vi "Programmatically Create SV.vi"(10 "database":path=path "C:/Ehsan Temp Folder/TFS/LV/Data Logging with LabVIEW/Database/FromDDS.csv" caption="Database (.csv) - \";\" separated", 11 "Project Address":path=path "C:/Ehsan Temp Folder/TFS/LV/Data Logging with LabVIEW/qq.lvproj") -> ()   [LabVIEW 2014]
uses:
  TypeDef/Q1 Create SV.ctl
  <vilib>/Utility/file.llb/Read From Spreadsheet File (string).vi
  <vilib>/Platform/browser.llb/Open URL in Default Browser (path).vi
  <vilib>/Utility/file.llb/Write To Spreadsheet File (string).vi
panel:
  in  "lib name":bool
  in  "Library Name":string="SV Library" caption="Library Name (Save As)"
  in  "save":bool
  in  "Bind":bool
  in  "Create":bool
  in  "exit":bool
  in  "initialize":bool
  out "Database":string[][](array[string])
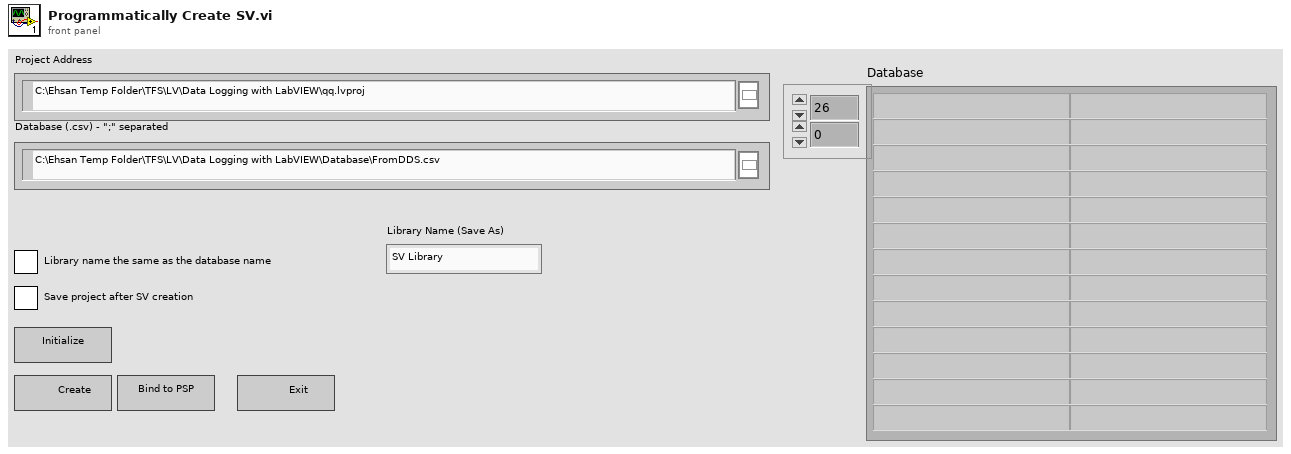
[diagram p1: front panel]
types:
  T1 = enum8{"Enabled", "Disabled", "Disabled and Grayed Out"}
  T2 = typedef "Q1 Create SV.ctl" = cluster{"State":enum16{"Initialize", "Idle", "Prepare", "Create", "Save Library", "Bind SV", "Exit", "Error", "Save Project", "Check Library Name"}, "Data":variant}
  T3 = enum16{"Initialize", "Idle", "Prepare", "Create", "Save Library", "Bind SV", "Exit", "Error", "Save Project", "Check Library Name"}
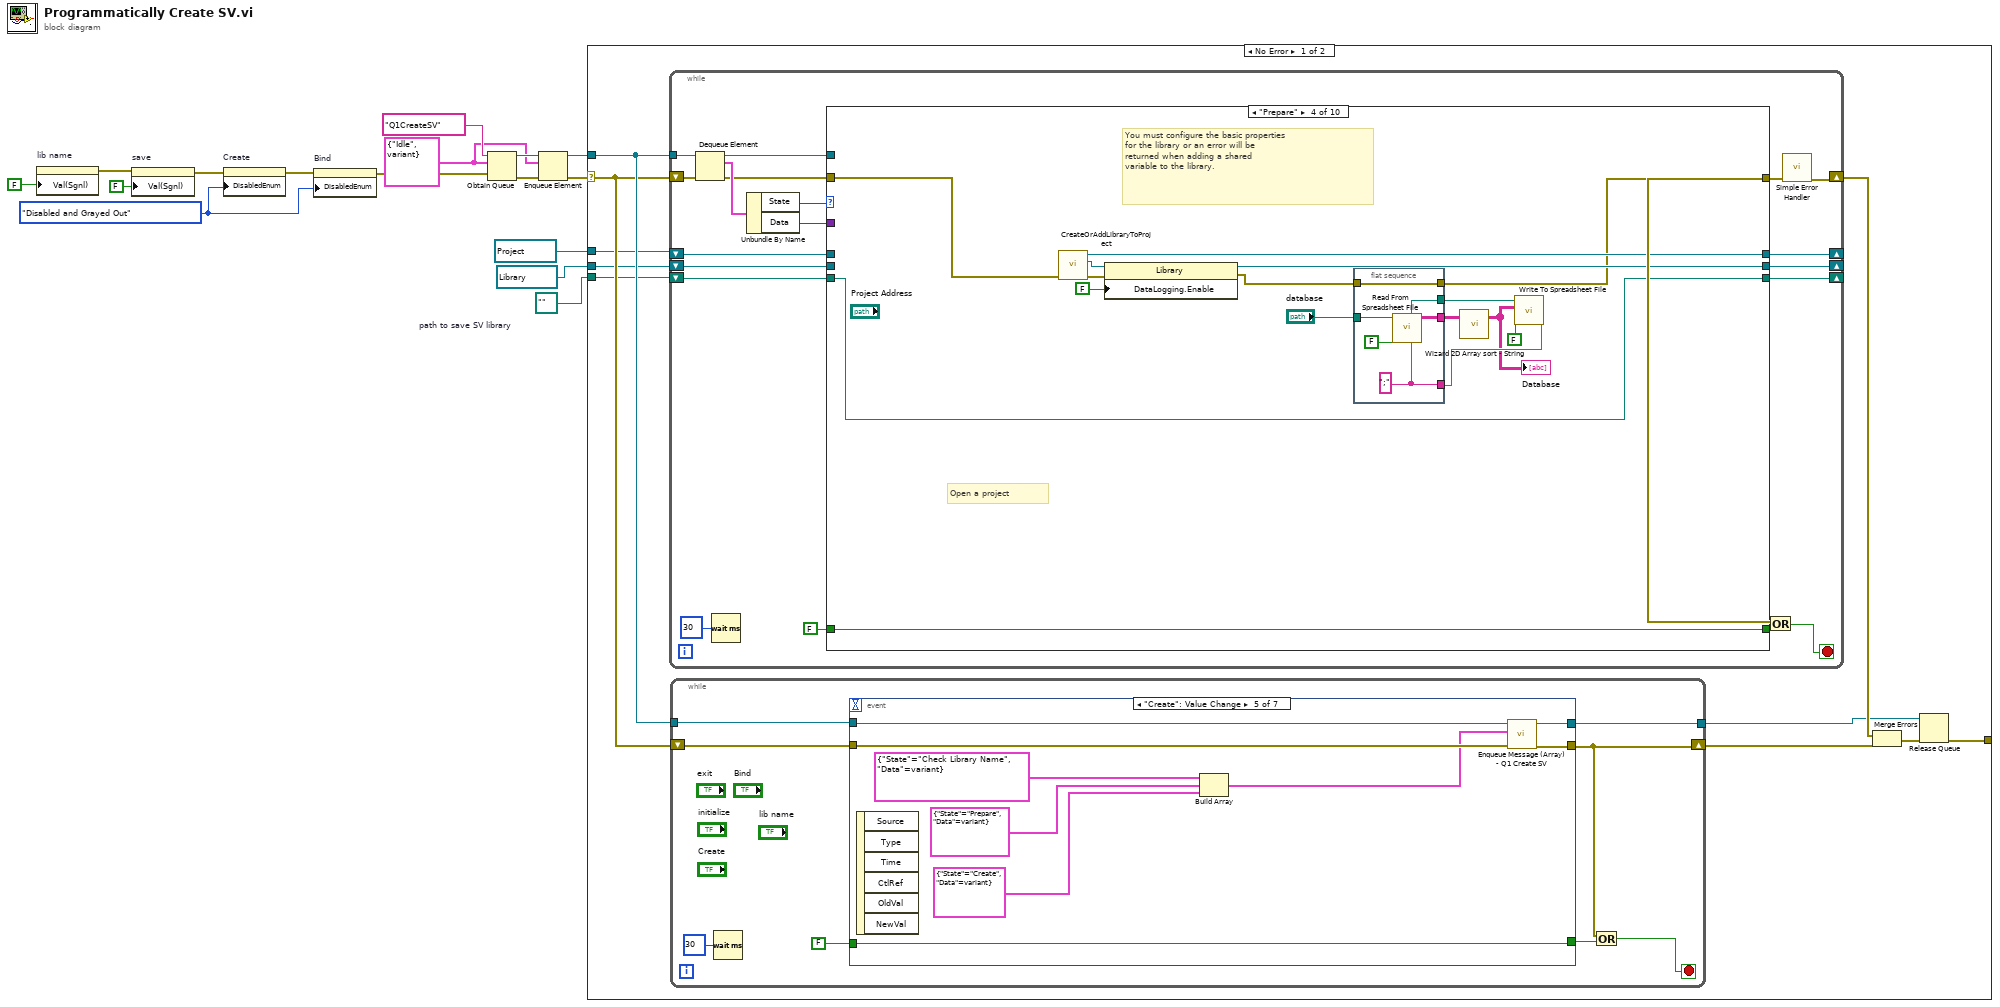
[diagram p0: block diagram]
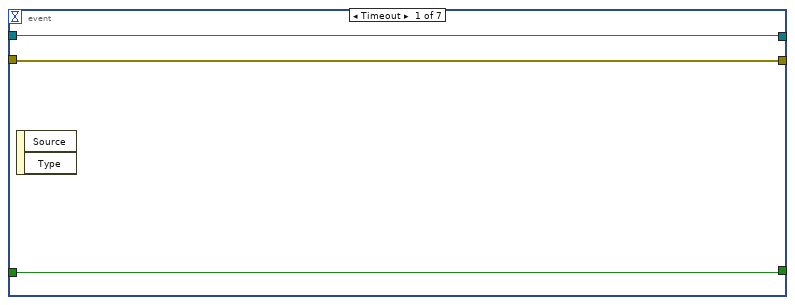
[diagram p2: hidden frame]
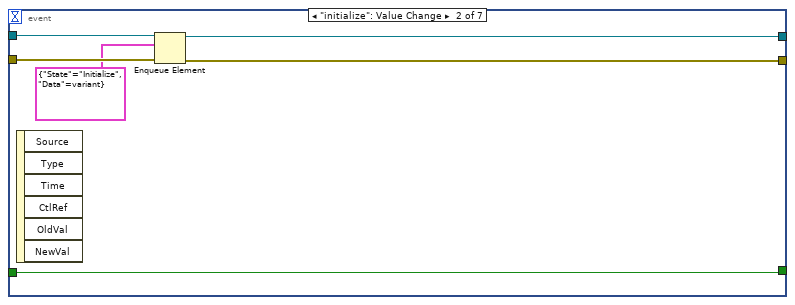
[diagram p3: hidden frame]
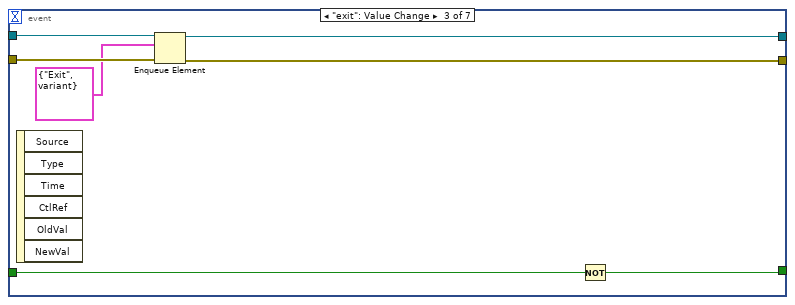
[diagram p4: hidden frame]
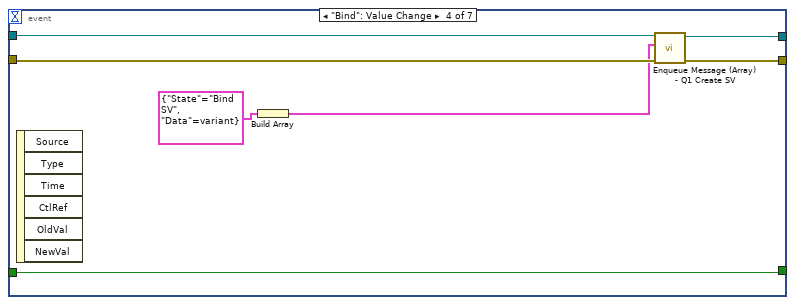
[diagram p5: hidden frame]
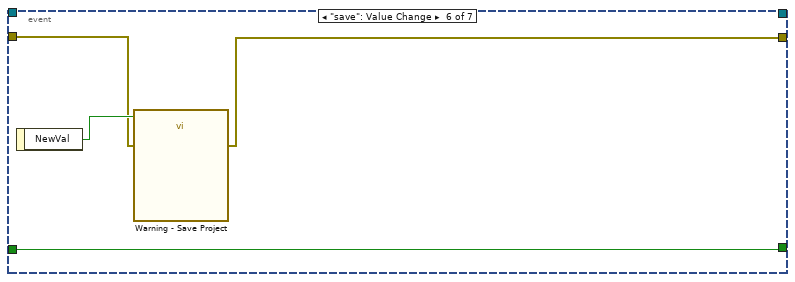
[diagram p6: hidden frame]
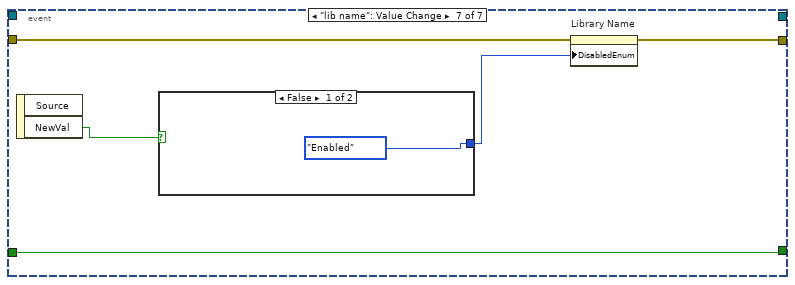
[diagram p7: hidden frame]
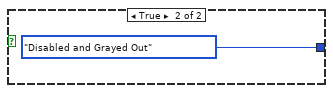
[diagram p8: hidden frame]
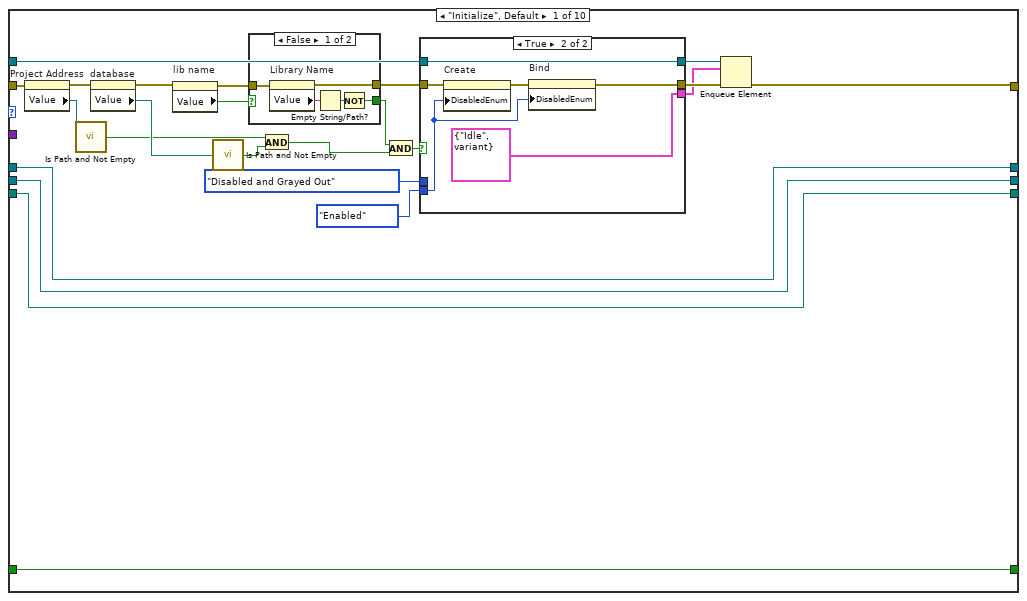
[diagram p9: hidden frame]
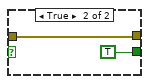
[diagram p10: hidden frame]
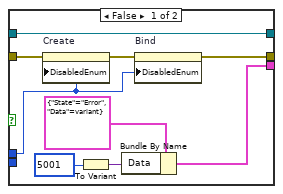
[diagram p11: hidden frame]
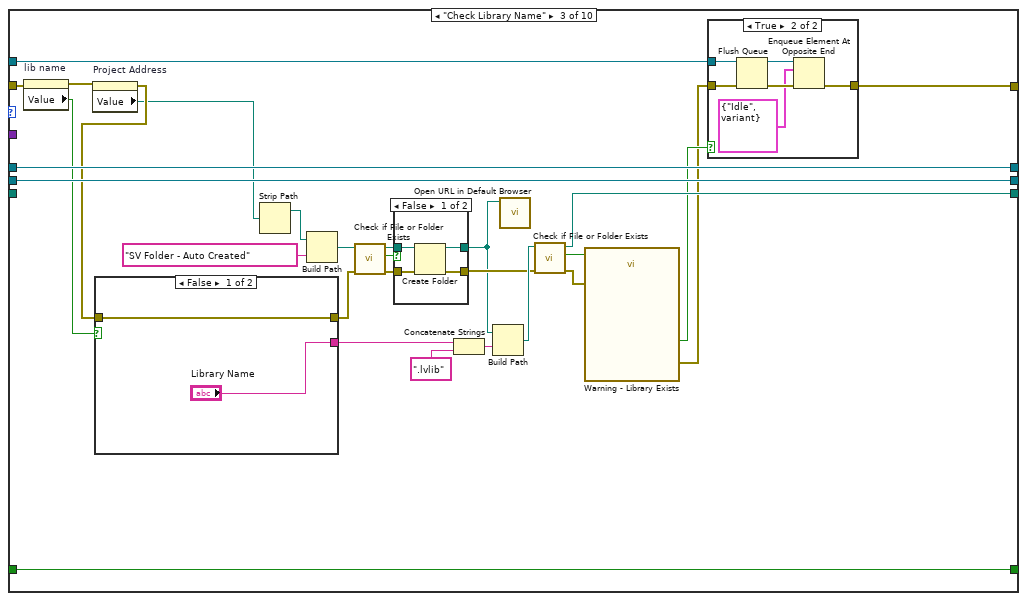
[diagram p13: hidden frame]
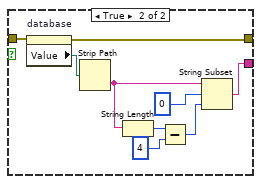
[diagram p14: hidden frame]
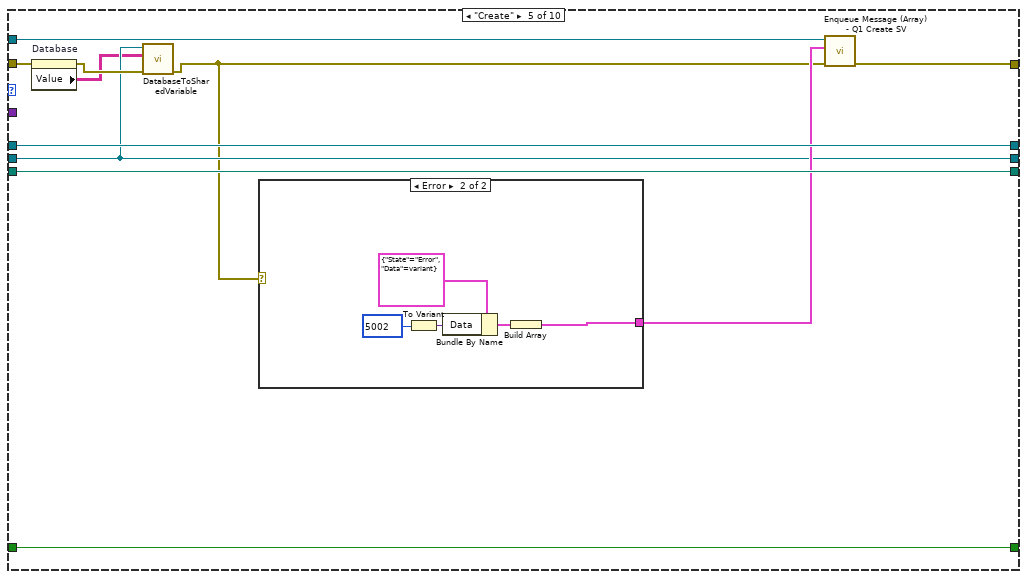
[diagram p17: hidden frame]
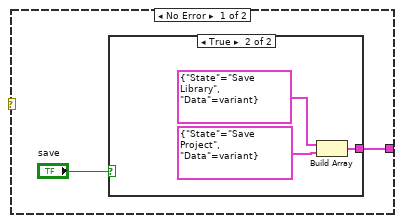
[diagram p18: hidden frame]
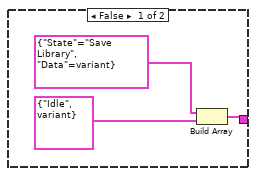
[diagram p19: hidden frame]
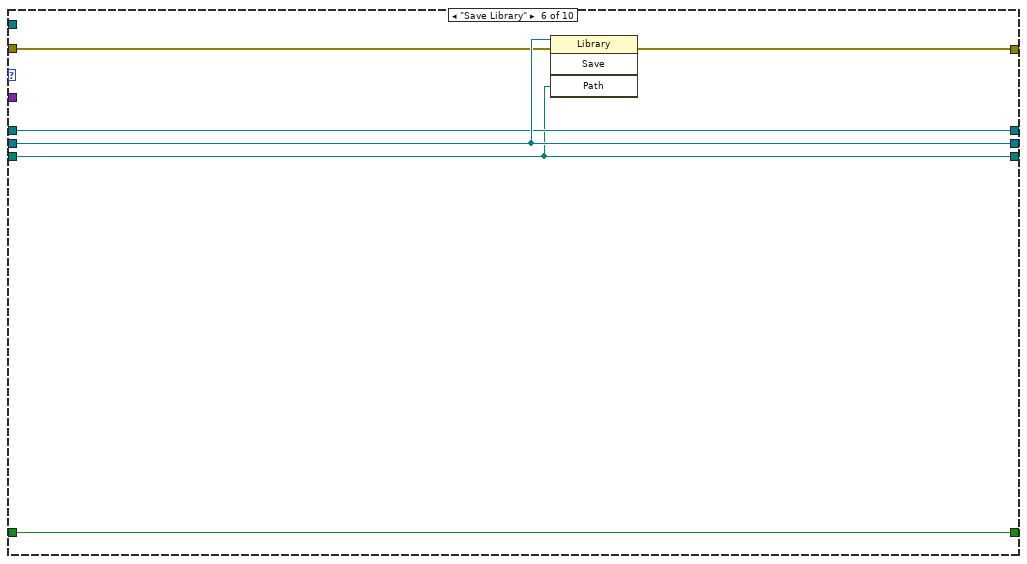
[diagram p20: hidden frame]
diagram:
  w6 = T1."Disabled and Grayed Out" ("Disabled")
  w8 = path ""  # path to save SV library
  w13 = T2 {"State"=enum."Idle", "Data"=variant}
  n1 = property on="lib name" class="Bool (strict)"("Val(Sgnl)"=FALSE ("Value (Signaling)")) -> (error out=w1:errorcluster)  [unwired: 2 in, 1 out]
  n2 = property on="save" class="Bool (strict)"(error in=w1, "Val(Sgnl)"=FALSE ("Value (Signaling)")) -> (error out=w4:errorcluster)  [unwired: 1 in, 1 out]
  n3 = property on="Create" class="Bool"(error in=w4, "DisabledEnum"=w6) -> (error out=w7:errorcluster)  [unwired: 1 in, 1 out]
  n4 = property on="Bind" class="Bool"(error in=w7, "DisabledEnum"=w6) -> (error out=w5:errorcluster)  [unwired: 1 in, 1 out]
  n5 = Obtain Queue(name (unnamed)="Q1CreateSV", element data type=w13, error in (no error)=w5) -> (queue out=w15:refnum<queue>, error out=w14:errorcluster)  [unwired: 2 in, 1 out]
  n6 = Enqueue Element(queue=w15, element=w13, error in (no error)=w14) -> (queue out=w11:refnum<queue>, error out=w12:errorcluster)  [unwired: 1 in, 1 out]
  n7 = case shown="No Error" w12 {
    selector: w12 -> [w25 w312]
    tunnel: w11 -> [w26 _]
    tunnel: refnum<vi> refnum ("Project Reference Out") -> [w24 _]
    tunnel: [w19 w312] -> _
    tunnel: refnum<vi> refnum ("Library Reference Out") -> [w18 _]
    tunnel: w8 -> [w17 _]
    frame No Error {
      n8 = while {
        tunnel: w26 -> [w95]
        shift-right: [w79] -> w22
        shift-left: w25 -> [w96]
        shift-right: [w86] -> _
        shift-left: w24 -> [w85]
        shift-right: [w84] -> _
        shift-left: w18 -> [w83]
        shift-right: [w82] -> _
        shift-left: w17 -> [w81]
        stop <- w88 stop-if-true
        n9 = Dequeue Element(queue=w95, error in (no error)=w96) -> (queue out=w91:refnum<queue>, element=w94:T2, error out=w80:errorcluster)  [unwired: 1 in, 1 out]
        n10 = Wait (ms)(milliseconds to wait=u32 30) -> ()  [unwired: 1 out]
        n11 = Unbundle By Name(w94) -> ("State"=w93:T3, "Data"=w92:variant)
        n12 = case shown="\"Prepare\"" w93 {
          tunnel: w92 -> [_ _ _ _ _ _ _ _ _ w310]
          tunnel: w91 -> [w108 _ w156 _ w229 _ _ w265 w290 w300]
          tunnel: FALSE -> [w120 w147 w175 w215 w232 w251 w259 w271 w289 w311]
          tunnel: [w120 w147 w175 w215 w232 w251 w259 w271 w288 w311] -> w89
          tunnel: [w105 w146 w174 w211 w231 w249 w255 w270 w279 w303] -> w86
          tunnel: w85 -> [w105 w146 w174 _ w231 w249 w255 w270 w279 w303]
          tunnel: [w104 w145 w173 w210 w224 w250 w256 w269 w284 w302] -> w84
          tunnel: w83 -> [w104 w145 w173 _ w224 w250 w256 w269 w284 w302]
          tunnel: [w103 w144 w160 w208 w230 w247 w258 w268 w287 w301] -> w82
          tunnel: w81 -> [w103 w144 _ w208 w230 w247 w258 w268 w287 w301]
          tunnel: [w102 w143 w157 w206 w227 w248 w253 w263 w286 w297] -> w78
          tunnel: w80 -> [w101 w143 w153 w202 w226 w246 w252 w261 w285 _]
          frame "Initialize", Default {
            n13 = property on="Project Address" class="Path"(error in=w101) -> (error out=w119:errorcluster, "Value"=w118:path)  [unwired: 1 in, 1 out]
            n14 = call <vilib>:"Is Path and Not Empty.vi"("path"=w118) -> ("Is Path and Not Empty?"=w115:bool)  [unwired: 4 in]
            n15 = property on="database" class="Path"(error in=w119) -> (error out=w100:errorcluster, "Value"=w117:path)  [unwired: 1 in, 1 out]
            n16 = property on="lib name" class="Bool (strict)"(error in=w100) -> (error out=w98:errorcluster, "Value"=w99:bool)  [unwired: 1 in, 1 out]
            n17 = call <vilib>:"Is Path and Not Empty.vi"("path"=w117) -> ("Is Path and Not Empty?"=w116:bool)  [unwired: 4 in]
            n18 = case shown="False" w99 {
              tunnel: [w124 TRUE] -> w114
              tunnel: w98 -> [w122 w127]
              tunnel: [w121 w127] -> w97
              frame False {
                n19 = property on="Library Name" class="Str"(error in=w122) -> (error out=w121:errorcluster, "Value"=w123:string)  [unwired: 1 in, 1 out]
                n20 = Empty String/Path?(string/path=w123) -> (empty?=w125:bool)
                n21 = Not(x=w125) -> (.not. x?=w124:bool)
              }
              frame True {
              }
            }
            n22 = And(x=w115, y=w116) -> (x .and. y?=w113:bool)
            n23 = And(x=w114, y=w113) -> (x .and. y?=w112:bool)
            n24 = case shown="True" w112 {
              tunnel: T1."Disabled and Grayed Out" ("Disabled") -> [w129 _]
              tunnel: T1."Enabled" ("Disabled") -> [_ w139]
              tunnel: [w133 T2 {"State"=enum."Idle", "Data"=variant}] -> w106
              tunnel: [w130 w138] -> w109
              tunnel: w108 -> [w132 w141]
              tunnel: [w132 w141] -> w107
              tunnel: w97 -> [w128 w137]
              frame False {
                n25 = property on="Create" class="Bool"(error in=w128, "DisabledEnum"=w129) -> (error out=w131:errorcluster)  [unwired: 1 in, 1 out]
                n26 = To Variant(anything=5001) -> (Variant=w134:variant)
                n27 = Bundle By Name(cluster=T2 {"State"=enum."Error", "Data"=variant}, "Data"=w134) -> (w133:T2)
                n28 = property on="Bind" class="Bool"(error in=w131, "DisabledEnum"=w129) -> (error out=w130:errorcluster)  [unwired: 1 in, 1 out]
              }
              frame True {
                n29 = property on="Create" class="Bool"(error in=w137, "DisabledEnum"=w139) -> (error out=w140:errorcluster)  [unwired: 1 in, 1 out]
                n30 = property on="Bind" class="Bool"(error in=w140, "DisabledEnum"=w139) -> (error out=w138:errorcluster)  [unwired: 1 in, 1 out]
              }
            }
            n31 = Enqueue Element(queue=w107, element=w106, error in (no error)=w109) -> (error out=w102:errorcluster)  [unwired: 1 in, 2 out]
          }
          frame "Idle" {
          }
          frame "Check Library Name" {
            n32 = property on="lib name" class="Bool (strict)"(error in=w153) -> (error out=w152:errorcluster, "Value"=w155:bool)  [unwired: 1 in, 1 out]
            n33 = property on="Project Address" class="Path"(error in=w152) -> (error out=w151:errorcluster, "Value"=w149:path)  [unwired: 1 in, 1 out]
            n34 = case shown="False" w155 {
              tunnel: ["Library Name" w183] -> w154
              tunnel: [w176 w185] -> w150
              tunnel: w151 -> [w176 w186]
              frame False {
              }
              frame True {
                n35 = property on="database" class="Path"(error in=w186) -> (error out=w185:errorcluster, "Value"=w184:path)  [unwired: 1 in, 1 out]
                n36 = Strip Path(path=w184) -> (name=w181:string)  [unwired: 1 out]
                n37 = String Length(string=w181) -> (length=w180:i32)
                n38 = Subtract(x=w180, y=4) -> (x-y=w178:i32)
                n39 = String Subset(string=w181, offset (0)=0, length (rest)=w178) -> (substring=w183:string)
              }
            }
            n40 = Strip Path(path=w149) -> (stripped path=w172:path)  [unwired: 1 out]
            n41 = Build Path(base path=w172, name or relative path="SV Folder - Auto Created") -> (appended path=w170:path)
            n42 = call <vilib>:"Check if File or Folder Exists.vi"("error in (no error)"=w150, "path"=w170) -> ("error out"=w169:errorcluster, "file or folder exists?"=w168:bool, "dup path"=w167:path)  [unwired: 7 in]
            n43 = case shown="False" w168 {
              tunnel: [w197 w198] -> w148
              tunnel: [w195 w199] -> w163
              tunnel: w169 -> [w196 w199]
              tunnel: w167 -> [w194 w198]
              frame False {
                n44 = Create Folder(path (use dialog)=w194, error in=w196) -> (created path=w197:path, error out=w195:errorcluster)  [unwired: 1 in, 1 out]
              }
              frame True {
              }
            }
            n45 = Concatenate Strings(w154, ".lvlib" ("string")) -> (w165:string)
            n46 = Build Path(base path=w148, name or relative path=w165) -> (appended path=w164:path)
            n47 = call-poly <vilib>:"Open URL in Default Browser.vi"("path"=w148) -> ()  [unwired: 5 in, 2 out]
            n48 = call <vilib>:"Check if File or Folder Exists.vi"("error in (no error)"=w163, "path"=w164) -> ("error out"=w162:errorcluster, "file or folder exists?"=w161:bool, "dup path"=w160:path)  [unwired: 7 in]
            n49 = call "Warning - Library Exists"("Enable"=w161, "error in (no error)"=w162) -> ("Stop"=w159:bool, "error out"=w158:errorcluster)  [unwired: 16 in]
            n50 = case shown="True" w159 {
              tunnel: [w187 w190] -> w157
              tunnel: w158 -> [w187 w189]
              tunnel: w156 -> [_ w188]
              frame False {
              }
              frame True {
                n51 = Flush Queue(queue=w188, error in (no error)=w189) -> (queue out=w193:refnum<queue>, error out=w192:errorcluster)  [unwired: 1 out]
                n52 = Enqueue Element At Opposite End(queue=w193, element=T2 {"State"=enum."Idle", "Data"=variant}, error in (no error)=w192) -> (error out=w190:errorcluster)  [unwired: 1 in, 2 out]
              }
            }
          }
          frame "Prepare" {
            # "Open a project"
            # "You must configure the basic properties\nfor the library or an error will be\nreturned when adding a shared\nvariable to the library."
            n53 = call <vilib>:"CreateOrAddLibraryToProject.vi"("error in (no error)"=w202) -> ("error out"=w213:errorcluster, "Library Reference Out"=w212:refnum<vi>, "Project Reference Out"=w211:refnum<vi>)  [unwired: 8 in]
            n54 = property class="Library"(reference=w212, error in=w213, "DataLogging.Enable"=FALSE ("DataLogging:Enable")) -> (reference out=w210:refnum<vi>, error out=w207:errorcluster)
            n55 = flat-sequence {
              tunnel: "database" -> [w220]
              tunnel: [w219] -> w201
              tunnel: w207 -> [w218]
              tunnel: [w218] -> w206
              tunnel: [w217] -> w205
              tunnel: [w216] -> w204
              frame #0 {
                w216 = ";" ("delimiter (\\t)")
                n56 = call-poly <vilib>:"Read From Spreadsheet File.vi"("delimiter (\\t)"=w216, "transpose (no:F)"=FALSE, "file path (dialog if empty)"=w220) -> ("all rows"=w219:string[][], "new file path (Not A Path if cancelled)"=w217:path)  [unwired: 4 in, 3 out]
              }
            }
            n57 = call "Wizard 2D Array sort - String.vi"("Array In"=w201) -> ("Array Out"=w200:string[][])  [unwired: 1 in, 1 out]
            "Database" <- w200
            n58 = call-poly <vilib>:"Write To Spreadsheet File.vi"("delimiter (\\t)"=w204, "append to file? (new file:F)"=FALSE, "2D data"=w200, "file path (dialog if empty)"=w205) -> ()  [unwired: 4 in, 1 out]
          }
          frame "Create" {
            n59 = property on="Database" class="Arr (strict)"(error in=w226) -> (error out=w225:errorcluster, "Value"=w223:string[][])  [unwired: 1 in, 1 out]
            n60 = call "DatabaseToSharedVariable.vi"("error in"=w225, 10:w223, "Library in"=w224) -> ("error out"=w222:errorcluster)  [unwired: 6 in, 2 out]
            n61 = case shown="Error" w222 {
              tunnel: [w234 w242] -> w228
              frame No Error {
                n62 = case shown="True" "save" {
                  tunnel: [w236 w238] -> w234
                  frame False {
                    n63 = Build Array(T2 {"State"=enum."Save Library", "Data"=variant}, T2 {"State"=enum."Idle", "Data"=variant}) -> (w236:T2[])
                  }
                  frame True {
                    n64 = Build Array(T2 {"State"=enum."Save Library", "Data"=variant}, T2 {"State"=enum."Save Project", "Data"=variant}) -> (w238:T2[])
                  }
                }
              }
              frame Error {
                n65 = To Variant(anything=5002) -> (Variant=w243:variant)
                n66 = Bundle By Name(cluster=T2 {"State"=enum."Error", "Data"=variant}, "Data"=w243) -> (w241:T2)
                n67 = Build Array(w241) -> (w242:T2[])
              }
            }
            n68 = call "Enqueue Message (Array) - Q1 Create SV.vi"("error in (no error)"=w222, "Message Array"=w228, "Qin"=w229) -> ("error out"=w227:errorcluster)  [unwired: 7 in, 1 out]
          }
          frame "Save Library" {
            n69 = invoke class="Library" method="Save"(reference=w250, error in=w246, "Path"=w247) -> (error out=w248:errorcluster)  [unwired: 1 in, 3 out]
          }
          frame "Save Project" {
            n70 = property on="Project Address" class="Path"(error in=w252) -> (error out=w254:errorcluster, "Value"=w257:path)  [unwired: 1 in, 1 out]
            n71 = invoke class="Project" method="Save"(reference=w255, error in=w254, "Path"=w257) -> (error out=w253:errorcluster)  [unwired: 1 in, 3 out]
          }
          frame "Bind SV" {
            n72 = property on="Database" class="Arr (strict)"(error in=w261) -> (error out=w267:errorcluster, "Value"=w260:string[][])  [unwired: 1 in, 1 out]
            n73 = call "BindingVI.vi"("Library Path"=w268, "error in"=w267, "Binding info"=w260) -> ("error out"=w266:errorcluster, "Error status"=w264:bool)  [unwired: 7 in]
            n74 = case shown="True" w264 {
              tunnel: [w272 w275] -> w262
              frame False {
                n75 = Build Array(T2 {"State"=enum."Idle", "Data"=variant}) -> (w272:T2[])
              }
              frame True {
                n76 = To Variant(anything=5003) -> (Variant=w276:variant)
                n77 = Bundle By Name(cluster=T2 {"State"=enum."Error", "Data"=variant}, "Data"=w276) -> (w274:T2)
                n78 = Build Array(w274) -> (w275:T2[])
              }
            }
            n79 = call "Enqueue Message (Array) - Q1 Create SV.vi"("error in (no error)"=w266, "Message Array"=w262, "Qin"=w265) -> ("error out"=w263:errorcluster)  [unwired: 7 in, 1 out]
          }
          frame "Exit" {
            n80 = Flush Queue(queue=w290, error in (no error)=w285) -> (error out=w280:errorcluster)  [unwired: 2 out]
            n81 = Not A Number/Path/Refnum?(number/path/refnum=w279) -> (NaN/Path/Refnum?=w283:bool)
            n82 = Not A Number/Path/Refnum?(number/path/refnum=w284) -> (NaN/Path/Refnum?=w282:bool)
            n83 = Or(x=w283, y=w282) -> (x .or. y?=w281:bool)
            n84 = case shown="True" w281 {
              tunnel: w284 -> [w295 _]
              tunnel: [w294 w296] -> w286
              tunnel: w280 -> [w293 w296]
              tunnel: w279 -> [w291 _]
              frame False {
                n85 = Close Reference(reference=w291, error in (no error)=w293) -> (error out=w292:errorcluster)
                n86 = Close Reference(reference=w295, error in (no error)=w292) -> (error out=w294:errorcluster)
              }
              frame True {
              }
            }
            n87 = Not(x=w289) -> (.not. x?=w288:bool)
          }
          frame "Error" {
            n88 = Variant To Data(type=0, Variant=w310) -> (data=w308:i32, error out=w304:errorcluster)  [unwired: 1 in]
            n89 = call <vilib>:"General Error Handler.vi"("[error code] (0)"=w308, "[user-defined codes]"=i32[] [5001, 5002, 5003], "[user-defined descriptions]"=string[] ["Error occured at Initialize state. Project Address and/or Database Address may not be a path or may be empty. The Library Name may be empty.\n", "Error occured in Create state. The type of the shared variable is not known to this SubVI. ", "Error occured at Bind state. There is something wrong with database (binding server, binding library name, SV name) or with the library that is to be bound."], "[error source] (\" \")"="Automatically Creation of Shared Variables" ("[error source] (\" \")"), "error in (no error)"=w304) -> ("error out"=w299:errorcluster)  [unwired: 6 in, 4 out]
            n90 = Enqueue Element(queue=w300, element=T2 {"State"=enum."Idle", "Data"=variant}, error in (no error)=w299) -> (error out=w297:errorcluster)  [unwired: 1 in, 2 out]
          }
        }
        n91 = Or(x=w78, y=w89) -> (x .or. y?=w88:bool)
        n92 = call <vilib>:"Simple Error Handler.vi"("error in (no error)"=w78) -> ("error out"=w79:errorcluster)  [unwired: 4 in, 4 out]
      }
      n93 = while {
        tunnel: w26 -> [w34]
        shift-right: [w29] -> w23
        shift-left: w25 -> [w33]
        tunnel: [w27] -> w20
        stop <- w30 stop-if-true
        n94 = Wait (ms)(milliseconds to wait=u32 30) -> ()  [unwired: 1 out]
        n95 = event shown="[4] \"Create\": Value Change" {
          selector: _ -> [_ _ _ _ _ _ _]
          dyn-events: _ -> [_ _ _ _ _ _ _]
          timeout: _ -> [_ _ _ _ _ _ _]
          tunnel: w34 -> [w36 w43 w50 w53 w62 _ _]
          tunnel: w33 -> [w35 w42 w49 w54 w61 w68 w73]
          tunnel: FALSE -> [w37 w40 w46 w57 w66 w70 w75]
          tunnel: [w37 w40 w45 w57 w66 w70 w75] -> w31
          tunnel: [w35 w39 w47 w55 w60 w67 w72] -> w29
          tunnel: [w36 w38 w44 w56 w63 _ _] -> w27
          event Timeout {
            n96 = event-data() -> ()  [unwired: 1 in, 2 out]
          }
          event "initialize": Value Change {
            n97 = event-data() -> ()  [unwired: 1 in, 6 out]
            n98 = Enqueue Element(queue=w43, element=T2 {"State"=enum."Initialize", "Data"=variant}, error in (no error)=w42) -> (queue out=w38:refnum<queue>, error out=w39:errorcluster)  [unwired: 1 in, 1 out]
          }
          event "exit": Value Change {
            n99 = event-data() -> ()  [unwired: 1 in, 6 out]
            n100 = Enqueue Element(queue=w50, element=T2 {"State"=enum."Exit", "Data"=variant}, error in (no error)=w49) -> (queue out=w44:refnum<queue>, error out=w47:errorcluster)  [unwired: 1 in, 1 out]
            n101 = Not(x=w46) -> (.not. x?=w45:bool)
          }
          event "Bind": Value Change {
            n102 = event-data() -> ()  [unwired: 1 in, 6 out]
            n103 = Build Array(T2 {"State"=enum."Bind SV", "Data"=variant}) -> (w51:T2[])
            n104 = call "Enqueue Message (Array) - Q1 Create SV.vi"("error in (no error)"=w54, "Message Array"=w51, "Qin"=w53) -> ("error out"=w55:errorcluster, "Qout"=w56:refnum<queue>)  [unwired: 7 in]
          }
          event "Create": Value Change {
            n105 = event-data() -> ()  [unwired: 1 in, 6 out]
            n106 = Build Array(T2 {"State"=enum."Check Library Name", "Data"=variant}, T2 {"State"=enum."Prepare", "Data"=variant}, T2 {"State"=enum."Create", "Data"=variant}) -> (w59:T2[])
            n107 = call "Enqueue Message (Array) - Q1 Create SV.vi"("error in (no error)"=w61, "Message Array"=w59, "Qin"=w62) -> ("error out"=w60:errorcluster, "Qout"=w63:refnum<queue>)  [unwired: 7 in]
          }
          event "save": Value Change {
            n108 = event-data() -> ("NewVal"=w69:bool)  [unwired: 1 in]
            n109 = call "Warning - Save Project"("Enable"=w69, "error in (no error)"=w68) -> ("error out"=w67:errorcluster)  [unwired: 16 in, 1 out]
          }
          event "lib name": Value Change {
            n110 = event-data() -> ("NewVal"=w74:bool)  [unwired: 1 in, 1 out]
            n111 = case shown="False" w74 {
              tunnel: [T1."Enabled" ("Disabled") T1."Disabled and Grayed Out" ("Disabled")] -> w71
              frame False {
              }
              frame True {
              }
            }
            n112 = property on="Library Name" class="Str"(error in=w73, "DisabledEnum"=w71) -> (error out=w72:errorcluster)  [unwired: 1 in, 1 out]
          }
        }
        n113 = Or(x=w29, y=w31) -> (x .or. y?=w30:bool)
      }
      n114 = Merge Errors(w22, w23) -> (w21:errorcluster)
      n115 = Release Queue(queue=w20, error in (no error)=w21) -> (error out=w19:errorcluster)  [unwired: 1 in, 2 out]
    }
    frame Error {
    }
  }
